vi "UART Get Bytes Available.vi"(8 "Error In":errorcluster, 10 "UART Channel":u8, 11 "LINX Device Config":T1) -> (0 "Error Out":errorcluster, 1 "Bytes Availabe":u8, 3 "LINX Device Config":T1)   [LabVIEW 2019, in "LMH-LINX.lvlib" / "Device.lvlib"]
doc: "Get the number of bytes available in the specified UART channel receive buffer."
uses:
  <vilib>/MakerHub/LINX/Private/Device/Device.lvlib
  <vilib>/MakerHub/LINX/Private/Device/Type Defs/LINX Device Config.ctl
  <vilib>/MakerHub/LINX/Private/Type Defs/Interface.ctl
  <vilib>/MakerHub/LINX/Private/Device/Type Defs/TCP Config.ctl
  <vilib>/MakerHub/LINX/Private/Device/Type Defs/Channels.ctl
  <vilib>/MakerHub/LINX/Private/Type Defs/Error Type.ctl
  <vilib>/MakerHub/LINX/LMH-LINX.lvlib
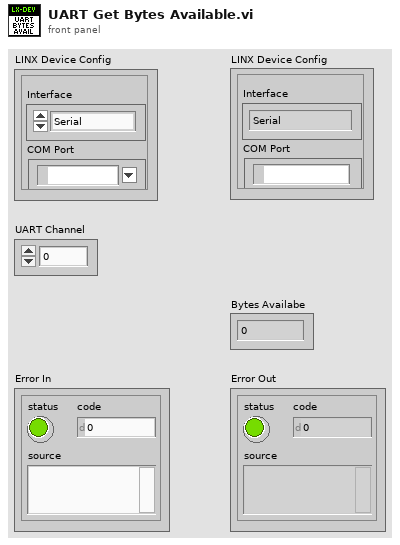
[diagram p1: front panel]
types:
  T1 = typedef "LMH-LINX.lvlib/Device.lvlib/LINX Device Config.ctl" = cluster{"Interface":T2, "COM Port":refnum<visa-resource-name>, "TCP Configuration":T3, "Device Family":u8, "Device ID":u8, "Device Name":string, "TCP Ref":refnum<k5>, "Channels":T4}
  T2 = typedef "LMH-LINX.lvlib/Interface.ctl" = enum16{"Serial", "TCP"}
  T3 = typedef "LMH-LINX.lvlib/Device.lvlib/TCP Config.ctl" = cluster{"IP Address":string, "Port":u16}
  T4 = typedef "LMH-LINX.lvlib/Channels.ctl" = cluster{"DI":u8[], "DO":u8[], "AI":u8[], "AO":u8[], "PWM":u8[], "QE":u8[], "UART":u8[], "I2C 2":u8[], "SPI":u8[], "CAN":u8[], "Servo":u8[], "AI Ref (V)":dbl, "AI Resolution (Bits)":u8, "AO Ref (V)":dbl, "AO Resolution (Bits)":u8}
  T5 = typedef "LMH-LINX.lvlib/Error Type.ctl" = enum16{"Unknown", "Timeout", "Corrupt Return Packet", "Unable To Connect", "Command Not Supported", "Channel DNE", "Invalid COM Config", "Firmware Version Mismatch", "myRIO Support", "CMD Specific Error", "Local IO Not Supported"}
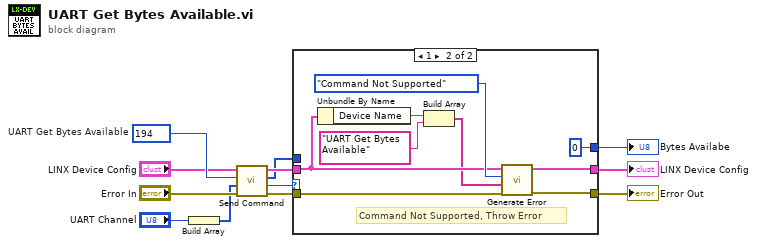
[diagram p0: block diagram]
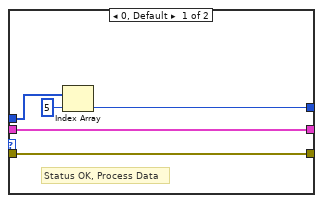
[diagram p2: hidden frame]
diagram:
  w11 = u16 194  # UART Get Bytes Available
  n1 = Build Array("UART Channel") -> (w4:u8[])
  n2 = call <vilib>:"Send Command.vi"("Error In"="Error In", "ARGS"=w4, "CMD"=w11, "LINX Device Config"="LINX Device Config") -> ("Error Out"=w6:errorcluster, "Status"=w1:u8, "Response"=w3:u8[], "LINX Device Config"=w8:T1)  [unwired: 4 in]
  n3 = case shown="1" w1 {
    tunnel: [w17 w24] -> w9
    tunnel: w8 -> [w17 w20]
    tunnel: [w16 w25] -> w7
    tunnel: w6 -> [w16 w26]
    tunnel: w3 -> [w15 _]
    tunnel: [w13 u8 0 ("element")] -> w2
    frame 0, Default {
      # "Status OK, Process Data"
      n4 = Index Array(array=w15, index=5) -> (element=w13:u8)
    }
    frame 1 {
      # "Command Not Supported, Throw Error"
      n5 = Unbundle By Name(w20) -> ("Device Name"=w22:string)
      n6 = Build Array(w22, "UART Get Bytes Available") -> (w19:string[])
      n7 = call <vilib>:"Generate Error.vi"("Error In"=w26, "Arguments"=w19, "Error Type"=Error_Type."Command Not Supported", "LINX Device Config"=w20) -> ("Error Out"=w25:errorcluster, "Dup LINX Device Config"=w24:T1)  [unwired: 6 in]
    }
  }
  "Error Out" <- w7
  "LINX Device Config" <- w9
  "Bytes Availabe" <- w2
